vi "PH_PSDBWriter.PC Set no PSDB Data collection.vi"(0 "i ref in":refnum<vi>, 5 "error IO":errorcluster) -> (14 "i ref out":refnum<vi>, 19 "error out":errorcluster)   [LabVIEW 2014, in "PH_PSDBWriter.lvlib"]
doc: "This VI sets the instance not to participate at the PSDB data collection."
uses:
  PH_PSDBWriter.lvlib
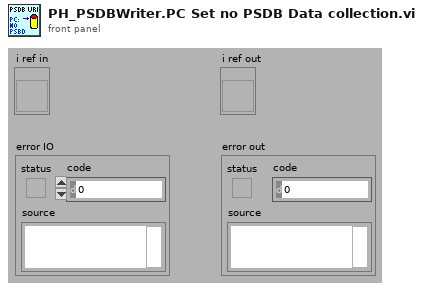
[diagram p1: front panel]
types:
  T1 = typedef "PH_PSDBWriter.lvlib/PH_PSDBWriter.i attribute.ctl" = cluster{"PSDB Status Service ID":i32, "Instance ID":i32, "Shot #":i32, "Subsystem":T2, "Data Status":T3, "Ref PSDB Status":refnum<vi>, "PSDB Error Code":i32, "PSDB Dataset":T4, "PSDB Thread":cluster{"Ref":refnum<vi>, "Q-Ref":refnum<queue>}, "PSDB Credentials":T12}
  T2 = typedef "PH_PSDBWriter.lvlib/PH_PSDBWriter.PHELIX-Subsystems.ctl" = i32
  T3 = typedef "PH_PSDBWriter.lvlib/PH_PSDBWriter.Data Status.ctl" = i16
  T4 = typedef "PH_PSDBWriter.lvlib/PH_PSDBWriter.PSDB Dataset.ctl" = cluster{"Version":i32, "2D data Input":T5[], "Boolean Input":T7[], "Image Input":T8[], "Numeric Input":T10[], "String Input":T11[]}
  T5 = typedef "PH_PSDBWriter.lvlib/PH_PSDBWriter.2D dataset.ctl" = cluster{"name":string, "data":dbl[][], "axis description":T6}
  T6 = typedef "PSDB.lvlib/PSDB_AxisDescription.ctl" = cluster{"x axis label":string, "y axis label":string, "x axis unit":string, "y axis unit":string}
  T7 = typedef "PH_PSDBWriter.lvlib/PH_PSDBWriter.Boolean dataset.ctl" = cluster{"name":string, "data":bool, "unit":string}
  T8 = typedef "PH_PSDBWriter.lvlib/PH_PSDBWriter.Image dataset.ctl" = cluster{"name":string, "data":T9, "unit":string}
  T9 = typedef "IMAQ Image.ctl" = refnum<image>
  T10 = typedef "PH_PSDBWriter.lvlib/PH_PSDBWriter.Numeric dataset.ctl" = cluster{"name":string, "data":dbl, "unit":string}
  T11 = typedef "PH_PSDBWriter.lvlib/PH_PSDBWriter.String dataset.ctl" = cluster{"name":string, "data":string, "unit":string}
  T12 = typedef "PH_Common.lvlib/PH_Connection.PSDB Credentials.ctl" = cluster{"PW":string, "ID":string, "DS":string}
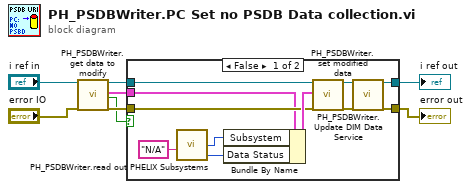
[diagram p0: block diagram]
diagram:
  n1 = call "PH_PSDBWriter.get data to modify.vi"("i ref in"="i ref in", "error in (no error)"="error IO") -> ("i ref out"=w2:refnum<vi>, "i attribute"=w4:T1, "timed out"=w1:bool, "error out"=w3:errorcluster)  [unwired: 14 in]
  n2 = case shown="False" w1 {
    tunnel: w3 -> [w16 w20]
    tunnel: w2 -> [w17 w21]
    tunnel: [w9 w20] -> w8
    tunnel: [w10 w21] -> w7
    tunnel: w4 -> [w13 _]
    frame False {
      n3 = call "PH_PSDBWriter.read out PHELIX Subsystems.vi"("Config DB Subsystem"="N/A") -> ("Metadata.Data Status"=w14:T3, "Metadata.Subsystem"=w18:T2)  [unwired: 2 in, 1 out]
      n4 = Bundle By Name(cluster=w13, "Subsystem"=w18, "Data Status"=w14) -> (w19:T1)
      n5 = call "PH_PSDBWriter.set modified data.vi"("i ref in"=w17, "i attribute"=w19, "error in (no error)"=w16) -> ("i ref out"=w11:refnum<vi>, "error out"=w12:errorcluster)  [unwired: 15 in]
      n6 = call "PH_PSDBWriter.Update DIM Data Service.vi"("i ref in"=w11, "error in"=w12) -> ("i ref out"=w10:refnum<vi>, "error out"=w9:errorcluster)  [unwired: 16 in]
    }
    frame True {
    }
  }
  "error out" <- w8
  "i ref out" <- w7
